vi "Main events.vi"(8 "error in (no error)":errorcluster, 11 "GUI Builder in":refnum<class "GUI Builder.lvclass">) -> (0 "error out":errorcluster, 3 "GUI Builder out":refnum<class "GUI Builder.lvclass">)   [LabVIEW 2021, in "App-Builder Library.lvlib" / "GUI Builder.lvclass"]
uses:
  GUI Builder.lvclass
  Builder/Builder.lvclass
panel:
  in  "Build all":bool
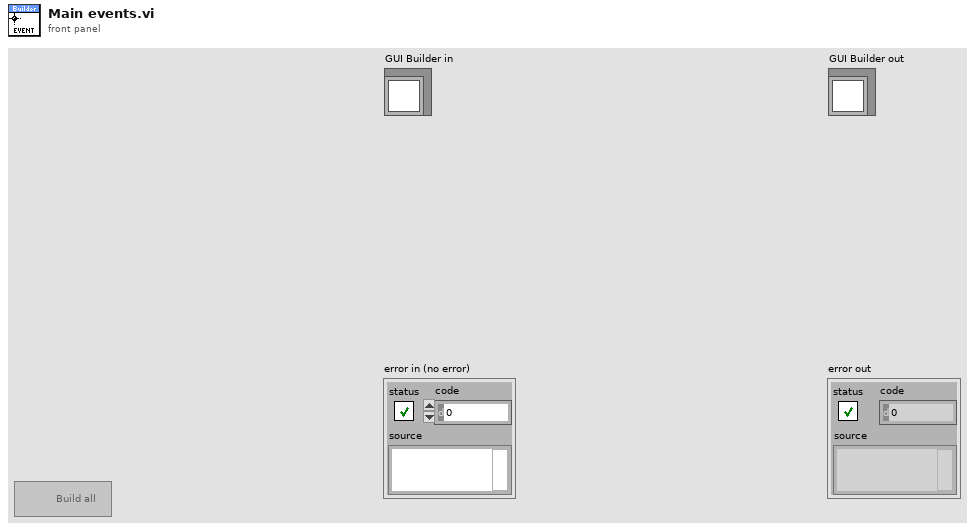
[diagram p1: front panel]
types:
  T1 = enum8{"Enabled", "Disabled", "Disabled and Grayed Out"}
  T2 = typedef "NI_App_Builder_API.lvlib/Build Specification Version.ctl" = cluster{"Major":u16, "Minor":u16, "Fix":u16, "Build":u16}
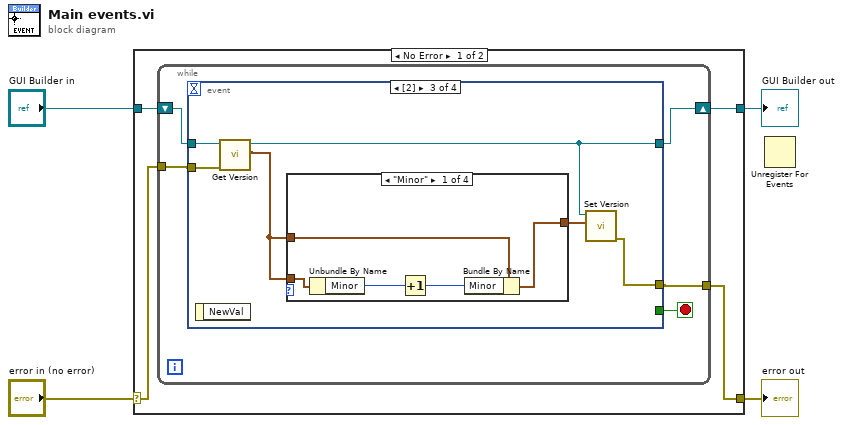
[diagram p0: block diagram]
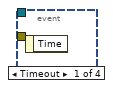
[diagram p2: hidden frame]
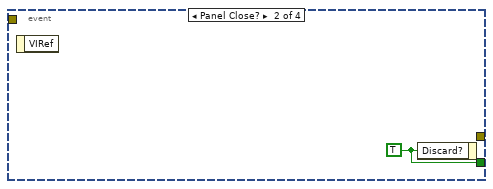
[diagram p3: hidden frame]
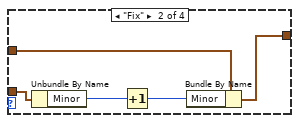
[diagram p4: hidden frame]
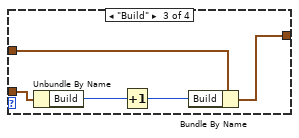
[diagram p5: hidden frame]
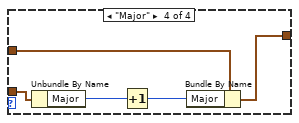
[diagram p6: hidden frame]
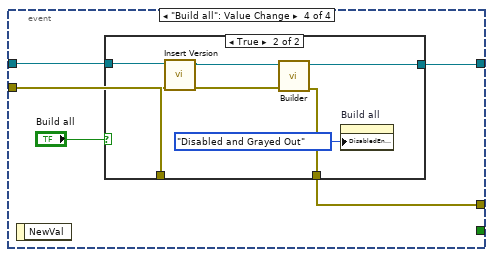
[diagram p7: hidden frame]
diagram:
  n1 = case shown="No Error" "error in (no error)" {
    selector: "error in (no error)" -> [w6 w56]
    tunnel: [w5 w56] -> w3
    tunnel: [w8 w55] -> w1
    tunnel: "GUI Builder in" -> [w7 w55]
    frame No Error {
      n2 = while {
        shift-right: [w13] -> w8
        shift-left: w7 -> [w12]
        tunnel: w6 -> [w11]
        tunnel: [w10] -> w5
        stop <- w9 stop-if-true
        n3 = event shown="[2]" {
          selector: _ -> [_ _ _ _]
          dyn-events: _ -> [_ _ _ _]
          timeout: _ -> [_ _ _ _]
          tunnel: [_ w14 _ _] -> w9
          tunnel: w12 -> [_ _ w20 w45]
          tunnel: [_ _ w19 w44] -> w13
          tunnel: [_ _ w16 w42] -> w10
          tunnel: w11 -> [_ _ w15 w43]
          event Timeout {
            n4 = event-data() -> ()  [unwired: 1 in, 1 out]
          }
          event Panel Close? {
            w14 = TRUE ("Discard?")
            n5 = event-data() -> ()  [unwired: 1 in, 1 out]
            n6 = event-data("Discard?"=w14) -> ()  [unwired: 1 in, 1 out]
          }
          event #2 (no event record) {
            n7 = event-data() -> ()  [unwired: 1 in, 1 out]
            n8 = call-dynamic "Get Version.vi"("error in (no error)"=w15, "Builder in"=w20) -> ("Build Version"=w17:T2, "Builder out"=w19:refnum<class "Builder.lvclass">)  [unwired: 7 in, 1 out]
            n9 = case shown="\"Minor\"" {
              selector: _ -> [_ _ _ _]
              tunnel: [w23 w28 w33 w38] -> w18
              tunnel: w17 -> [w25 w30 w35 w40]
              tunnel: w17 -> [w24 w29 w34 w39]
              frame "Minor" {
                n10 = Unbundle By Name(w25) -> ("Minor"=w22:u16)
                n11 = Increment(x=w22) -> (x+1=w21:u16)
                n12 = Bundle By Name(cluster=w24, "Minor"=w21) -> (w23:T2)
              }
              frame "Fix" {
                n13 = Unbundle By Name(w30) -> ("Minor"=w27:u16)
                n14 = Increment(x=w27) -> (x+1=w26:u16)
                n15 = Bundle By Name(cluster=w29, "Minor"=w26) -> (w28:T2)
              }
              frame "Build" {
                n16 = Unbundle By Name(w35) -> ("Build"=w32:u16)
                n17 = Increment(x=w32) -> (x+1=w31:u16)
                n18 = Bundle By Name(cluster=w34, "Build"=w31) -> (w33:T2)
              }
              frame "Major" {
                n19 = Unbundle By Name(w40) -> ("Major"=w37:u16)
                n20 = Increment(x=w37) -> (x+1=w36:u16)
                n21 = Bundle By Name(cluster=w39, "Major"=w36) -> (w38:T2)
              }
            }
            n22 = call "Set Version.vi"("Build Version"=w18, "Builder in"=w19) -> ("error out"=w16:errorcluster)  [unwired: 8 in, 1 out]
          }
          event "Build all": Value Change {
            n23 = event-data() -> ()  [unwired: 1 in, 1 out]
            n24 = case shown="True" "Build all" {
              tunnel: w45 -> [w46 w49]
              tunnel: [w46 w54] -> w44
              tunnel: w43 -> [w47 w48]
              tunnel: [w47 w53] -> w42
              frame False {
              }
              frame True {
                n25 = call "Insert Version.vi"("error in (no error)"=w48, "Builder in"=w49) -> ("error out"=w51:errorcluster, "Builder out"=w50:refnum<class "Builder.lvclass">)  [unwired: 8 in]
                n26 = call "Builder.vi"("error in"=w51, "Builder in"=w50) -> ("error out"=w53:errorcluster, "Builder out"=w54:refnum<class "Builder.lvclass">)  [unwired: 7 in, 1 out]
                n27 = property on="Build all" class="Bool"("DisabledEnum"=T1."Disabled and Grayed Out" ("Disabled")) -> ()  [unwired: 2 in, 2 out]
              }
            }
          }
        }
      }
    }
    frame Error {
    }
  }
  "error out" <- w3
  "GUI Builder out" <- w1
  n28 = Unregister For Events() -> ()  [unwired: 2 in, 1 out]
